vi "GetRefs.vi"(8 "error in (no error)":errorcluster, 11 "panel":refnum<vi>) -> (0 "error out":errorcluster, 3 "Refs":refnum<vi>[](array[refnum]))   [LabVIEW 2017]
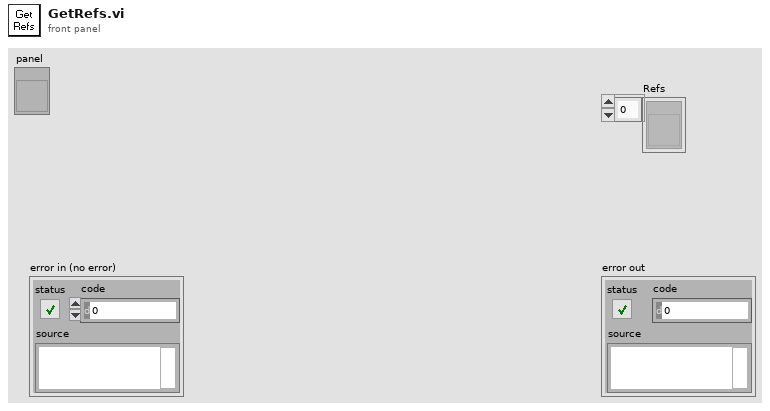
[diagram p1: front panel]
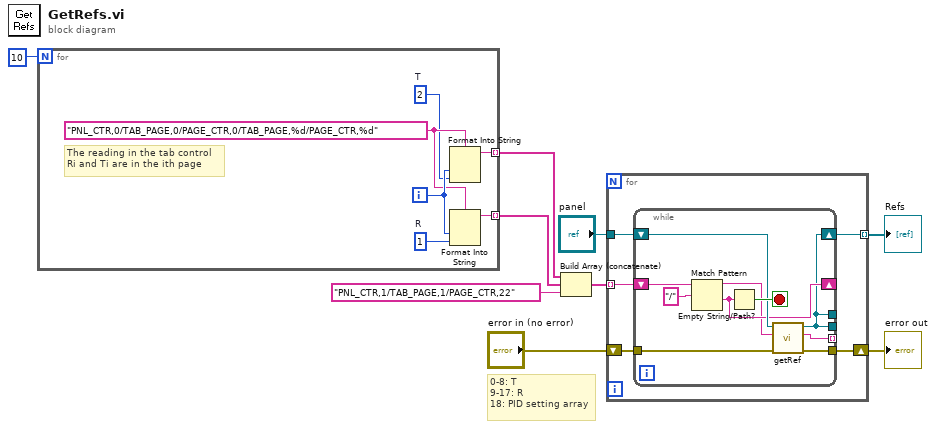
[diagram p0: block diagram]
diagram:
  # "0-8: T\n9-17: R\n18: PID setting array"
  n1 = for {
    N: 10 -> [_]
    tunnel: [w13] -> w3 mode=indexing
    tunnel: [w10] -> w4 mode=indexing
    i -> [w15]
    w11 = 1  # R
    w12 = 2  # T
    w14 = "PNL_CTR,0/TAB_PAGE,0/PAGE_CTR,0/TAB_PAGE,%d/PAGE_CTR,%d"
    # "The reading in the tab control\nRi and Ti are in the ith page"
    n2 = Format Into String(format string=w14, w15, w12) -> (resulting string=w13:string)  [unwired: 2 in, 1 out]
    n3 = Format Into String(format string=w14, w15, w11) -> (resulting string=w10:string)  [unwired: 2 in, 1 out]
  }
  n4 = Build Array (concatenate)(w3, w4, "PNL_CTR,1/TAB_PAGE,1/PAGE_CTR,22") -> (w1:string[])
  n5 = for {
    shift-right: [w19] -> w8
    shift-left: "error in (no error)" -> [w20]
    tunnel: [w18] -> w9 mode=indexing
    tunnel: "panel" -> [w17]
    tunnel: w1 -> [w16] mode=indexing
    n6 = while {
      shift-right: [w26] -> _
      shift-left: w16 -> [w30]
      shift-right: [w21] -> w18
      shift-left: w17 -> [w27]
      tunnel: w20 -> [w25]
      tunnel: [w24] -> w19
      tunnel: [w21] -> _
      tunnel: [w22] -> _ mode=indexing
      tunnel: [w21] -> _
      stop <- w28 stop-if-true
      n7 = Match Pattern(string=w30, regular expression="/" ("搜索字符串/字符(-)")) -> (before substring=w23:string, after substring=w26:string)  [unwired: 3 out]
      n8 = Empty String/Path?(string/path=w26) -> (empty?=w28:bool)
      n9 = call "getRef.vi"("Error out"=w25, "Name"=w23, "Gen ref in"=w27) -> ("Error out"=w24:errorcluster, "Cousins"=w22:string, "Gen ref out"=w21:refnum<vi>)  [unwired: 6 in]
    }
  }
  "Refs" <- w9
  "error out" <- w8
